vi "Vision Processing.vi"(4 "error in (no error)":errorcluster, 7 "Image Size":T1=enum."160x120") -> ()   [LabVIEW 2017]
doc: "This VI runs in parallel to other tasks. It gets images from the camera, processes them for color or shape and use that information to affect robot behavior."
uses:
  <vilib>/Rock Robotics/WPI/Camera/WPI_CameraImageSize.ctl
  <vilib>/Rock Robotics/WPI/Camera/WPI_CameraWhite Balance Values.ctl
  <vilib>/Rock Robotics/WPI/Camera/WPI_CameraExposure Values.ctl
  <vilib>/Rock Robotics/WPI/Camera/WPI_CameraFrameRate.ctl
  Robot Global Data.vi
  <vilib>/vision/NI_Vision_Development_Module.lvlib
panel:
  out "ParticleArea":dbl
  in  "Lum":cluster{"Lower value":i32, "Upper value":i32}={"Lower value"=30, "Upper value"=100}
  in  "Sat":cluster{"Lower value":i32, "Upper value":i32}={"Lower value"=130, "Upper value"=255}
  in  "Hue":cluster{"Lower value":i32, "Upper value":i32}={"Lower value"=70, "Upper value"=130}
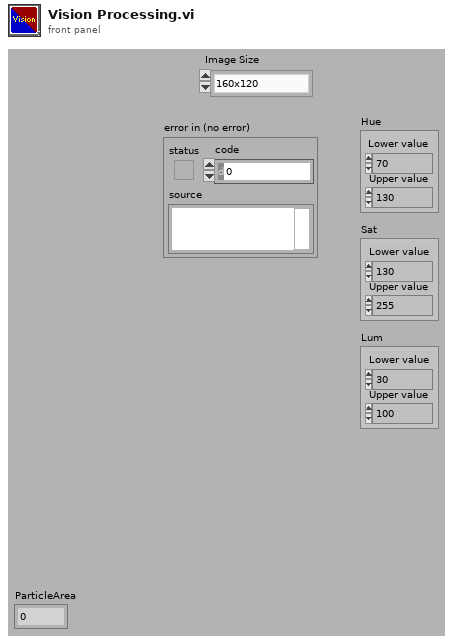
[diagram p1: front panel]
types:
  T1 = typedef "WPI_CameraImageSize.ctl" = enum16{"640x480", "320x240", "160x120", "Custom"}
  T2 = typedef "WPI_CameraFrameRate.ctl" = u32
  T3 = typedef "WPI_CameraExposure Values.ctl" = enum16{"Auto", "Flicker-free 50 Hz", "Flicker-free 60 Hz", "Hold current", "Custom"}
  T4 = typedef "WPI_CameraWhite Balance Values.ctl" = enum16{"Auto", "Fixed indoor", "Fixed outdoor 1", "Fixed outdoor 2", "Fixed fluorescent 1", "Fixed fluorescent 2", "Hold current", "Custom"}
  T5 = typedef "WPI_CameraDevRef.ctl" = cluster{"Camera Address":string, "CameraStatus":errorcluster}
  T6 = typedef "IMAQ Image.ctl" = refnum<image>
  T7 = typedef "Particle Parameters" = i32
  T8 = cluster{"Measurement Parameter":T7, "Range Lower Value":dbl, "Range Upper Value":dbl, "Range":bool, "Measurement Type":bool}[]
  T9 = typedef "Image Type" = u32
  T10 = cluster{"Area":dbl, "Number of Holes":dbl, "Bounding Rect":cluster{"Left":dbl, "Top":dbl, "Right":dbl, "Bottom":dbl}, "Center of Mass":cluster{"X":dbl, "Y":dbl}, "Orientation":dbl, "Dimensions":cluster{"Width":dbl, "Height":dbl}}[]
  T11 = cluster{"Area":dbl, "Number of Holes":dbl, "Bounding Rect":cluster{"Left":dbl, "Top":dbl, "Right":dbl, "Bottom":dbl}, "Center of Mass":cluster{"X":dbl, "Y":dbl}, "Orientation":dbl, "Dimensions":cluster{"Width":dbl, "Height":dbl}}
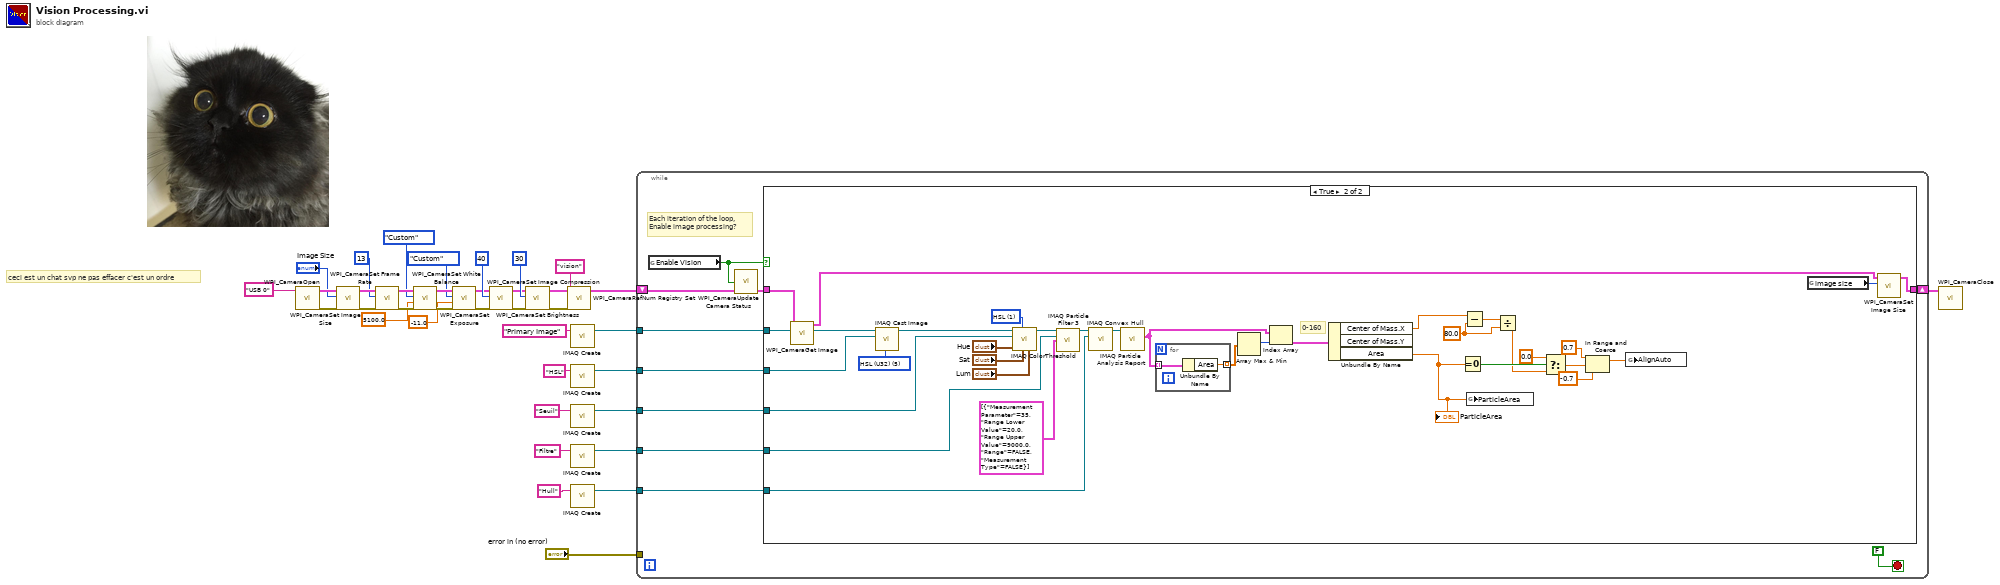
[diagram p0: block diagram]
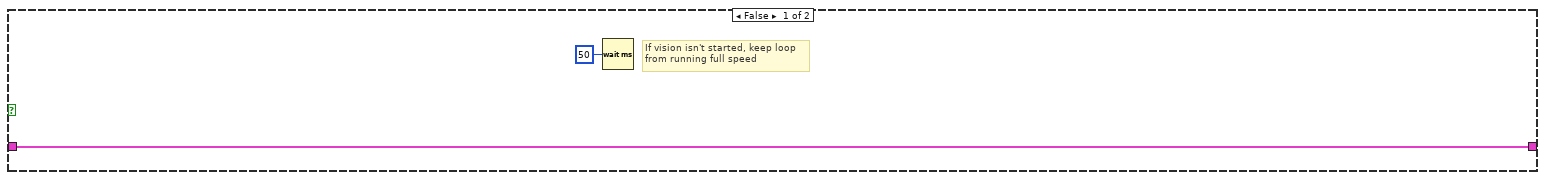
[diagram p2: hidden frame]
diagram:
  # "ceci est un chat svp ne pas effacer c'est un ordre"
  n1 = call <vilib>:"WPI_CameraOpen.vi"("Camera Address"="USB 0" ("format string")) -> ("error out"=w26:errorcluster, "CameraDevRef"=w27:T5)  [unwired: 1 in, 8 out]
  n2 = call <vilib>:"WPI_CameraSet Image Size.vi"("error in (no error)"=w26, "Image Size"="Image Size", "CameraDevRef"=w27) -> ("error out"=w25:errorcluster, "CameraDevRef Out"=w28:T5)  [unwired: 1 in, 6 out]
  n3 = call <vilib>:"WPI_CameraSet Frame Rate.vi"("error in (no error)"=w25, "Frame Rate (fps)"=T2 13, "CameraDevRef"=w28) -> ("error out"=w24:errorcluster, "CameraDevRef Out"=w30:T5)  [unwired: 7 out]
  n4 = call <vilib>:"WPI_CameraSet White Balance.vi"("error in (no error)"=w24, "Color Temp (K)"=5100.0, "White Balance"=WPI_CameraWhite_Balance_Values."Custom", "CameraDevRef"=w30) -> ("error out"=w23:errorcluster, "CameraDevRef Out"=w29:T5)  [unwired: 6 out]
  n5 = call <vilib>:"WPI_CameraSet Exposure.vi"("error in (no error)"=w23, "Exposure (%)"=-11.0, "Exposure"=WPI_CameraExposure_Values."Custom", "CameraDevRef"=w29) -> ("error out"=w22:errorcluster, "CameraDevRef Out"=w32:T5)  [unwired: 6 out]
  n6 = call <vilib>:"WPI_CameraSet Image Compression.vi"("error in (no error)"=w22, "Compression"=40, "CameraDevRef"=w32) -> ("error out"=w21:errorcluster, "CameraDevRef Out"=w31:T5)  [unwired: 7 out]
  n7 = call <vilib>:"WPI_CameraSet Brightness.vi"("error in (no error)"=w21, "Brightness"=30, "CameraDevRef"=w31) -> ("error out"=w19:errorcluster, "CameraDevRef Out"=w20:T5)  [unwired: 1 in, 6 out]
  n8 = call <vilib>:"WPI_CameraRefNum Registry Set.vi"("error in (no error)"=w19, "refnum name"="vision", "CameraDevRef"=w20) -> ("CameraDevRef"=w15:T5)  [unwired: 1 in, 7 out]
  n9 = call "IMAQ Create"("Image Name"="Primary Image") -> ("New Image"=w36:T6)  [unwired: 3 in, 2 out]
  n10 = call "IMAQ Create"("Image Name"="HSL") -> ("New Image"=w4:T6)  [unwired: 3 in, 2 out]
  n11 = call "IMAQ Create"("Image Name"="Seuil") -> ("New Image"=w3:T6)  [unwired: 3 in, 2 out]
  n12 = call "IMAQ Create"("Image Name"="Filtre") -> ("New Image"=w2:T6)  [unwired: 3 in, 2 out]
  n13 = call "IMAQ Create"("Image Name"="Hull") -> ("New Image"=w1:T6)  [unwired: 3 in, 2 out]
  n14 = while {
    shift-right: [w46] -> w13
    shift-left: w15 -> [w44]
    tunnel: w36 -> [w45]
    tunnel: "error in (no error)" -> [_]
    tunnel: w4 -> [w41]
    tunnel: w3 -> [w40]
    tunnel: w2 -> [w39]
    tunnel: w1 -> [w38]
    stop <- FALSE stop-if-true
    # "Each iteration of the loop,\nEnable image processing?"
    n15 = global read "Robot Global Data.vi" "Enable Vision"() -> (w42:bool)
    n16 = call <vilib>:"WPI_CameraUpdate Camera Status.vi"("CameraDevRef In"=w44, "Enable Vision"=w42) -> ("CameraDevRef Out"=w43:T5)  [unwired: 3 in]
    n17 = case shown="True" w42 {
      tunnel: w45 -> [_ w71]
      tunnel: [w49 w84] -> w46
      tunnel: w43 -> [w49 w82]
      tunnel: w41 -> [_ w69]
      tunnel: w40 -> [_ w67]
      tunnel: w39 -> [_ w66]
      tunnel: w38 -> [_ w65]
      frame False {
        # "If vision isn't started, keep loop\nfrom running full speed"
        n18 = Wait (ms)(milliseconds to wait=u32 50) -> ()  [unwired: 1 out]
      }
      frame True {
        w60 = 80.0 ("y")
        w70 = u16 1 items=["RGB", "HSL", "HSV", "HSI"] ("Color Mode")
        w68 = T9 5 items=["Grayscale (U8)", "Grayscale (I16)", "Grayscale (SGL)", "Complex (CSG)", "RGB (U32)", "HSL (U32)", "RGB (U64)", "Grayscale (U16)"] ("Image Type")
        # "0-160"
        n19 = call <vilib>:"WPI_CameraGet Image.vi"("Image"=w71, "CameraDevRef"=w82) -> ("Image Out"=w72:T6, "CameraDevRef Out"=w81:T5)  [unwired: 1 in, 7 out]
        n20 = call "IMAQ Cast Image"("Image Type"=w68, "Image Dst"=w69, "Image Src"=w72) -> ("Image Dst Out"=w73:T6)  [unwired: 7 in, 1 out]
        n21 = call "IMAQ ColorThreshold"("Blue or Luma or Val or Inten Range"="Lum", "Green or Sat Range"="Sat", "Color Mode"=w70, "Red or Hue Range"="Hue", "Image Dst"=w67, "Image Src"=w73) -> ("Image Dst Out"=w77:T6)  [unwired: 4 in, 1 out]
        n22 = call "IMAQ Particle Filter 3"("Image Src"=w77, "Image Dst"=w66, "Selection Values"=T8 [{"Measurement Parameter"=35, "Range Lower Value"=20.0, "Range Upper Value"=9000.0, "Range"=FALSE, "Measurement Type"=FALSE}]) -> ("Image Dst Out"=w74:T6)  [unwired: 10 in, 2 out]
        n23 = call "IMAQ Convex Hull"("Image Dst"=w65, "Image Src"=w74) -> ("Image Dst Out"=w75:T6)  [unwired: 8 in, 1 out]
        n24 = call "IMAQ Particle Analysis Report"("Image"=w75) -> ("Particle Reports (Pixels)"=w63:T10)  [unwired: 5 in, 5 out]
        n25 = for {
          tunnel: w63 -> [w86] mode=indexing
          tunnel: [w85] -> w64 mode=indexing
          n26 = Unbundle By Name(w86) -> ("Area"=w85:dbl)
        }
        n27 = Array Max & Min(array=w64) -> (max index (indices)=w62:i32)  [unwired: 3 out]
        n28 = Index Array(array=w63, index=w62) -> (element=w51:T11)
        n29 = Unbundle By Name(w51) -> ("Center of Mass.X"=w50:dbl, "Area"=w59:dbl)  [unwired: 1 out]
        "ParticleArea" <- w59
        n30 = Equal To 0?(x=w59) -> (x = 0?=w58:bool)
        n31 = Subtract(x=w50, y=w60) -> (x-y=w61:dbl)
        n32 = global write "Robot Global Data.vi" "ParticleArea"(w59) -> ()
        n33 = Divide(x=w61, y=w60) -> (x/y=w57:dbl)
        n34 = Select(t=0.0, s=w58, f=w57) -> (s? t:f=w55:dbl)
        n35 = In Range and Coerce(upper limit=0.7, x=w55, lower limit=-0.7) -> (coerced(x)=w54:dbl)  [unwired: 1 out]
        n36 = global write "Robot Global Data.vi" "AlignAuto"(w54) -> ()
        n37 = global read "Robot Global Data.vi" "image size"() -> (w83:T1)
        n38 = call <vilib>:"WPI_CameraSet Image Size.vi"("Image Size"=w83, "CameraDevRef"=w81) -> ("CameraDevRef Out"=w84:T5)  [unwired: 2 in, 7 out]
      }
    }
  }
  n39 = call <vilib>:"WPI_CameraClose.vi"("CameraDevRef"=w13) -> ()  [unwired: 1 in, 10 out]
